vi "FitterParams.vi"(7 "eTestType":T1(ring), 8 "error in (no error)":errorcluster, 10 "SignalParams":dbl[][](array[numeric])) -> (0 "error out":errorcluster, 2 "FitterParams":dbl[](array[numeric]))   [LabVIEW 2018, in "AnalysisPlugins.lvlib" / "PmuAnalysis.lvclass"]
uses:
  PmuAnalysis.lvclass
  <vilib>/Utility/error.llb/Error Cluster From Error Code.vi
  <vilib>/ErrorRing/Error Ring.xnode
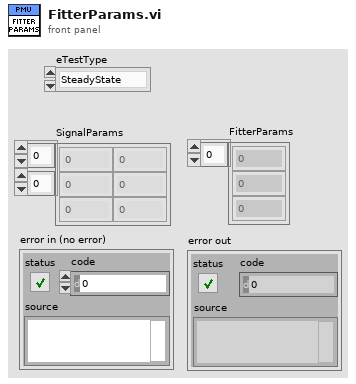
[diagram p1: front panel]
types:
  T1 = enum16{"SteadyState", "Modulation", "Ramp", "Step"}
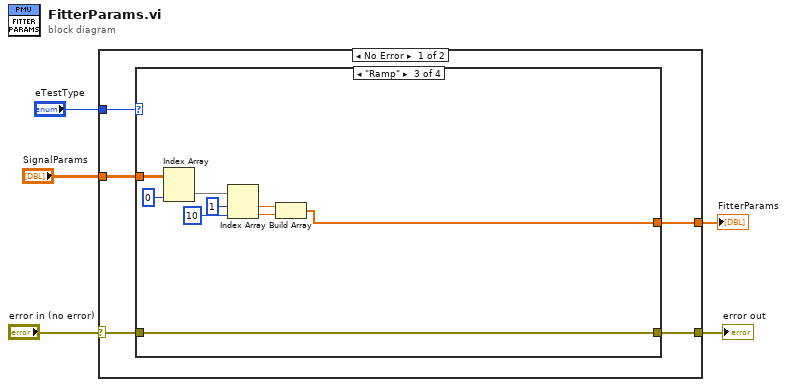
[diagram p0: block diagram]
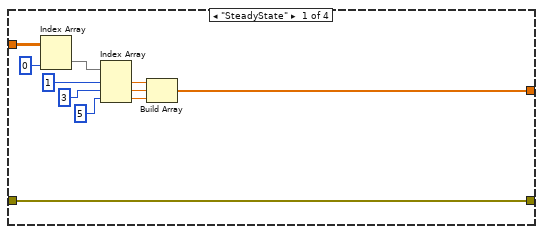
[diagram p2: hidden frame]
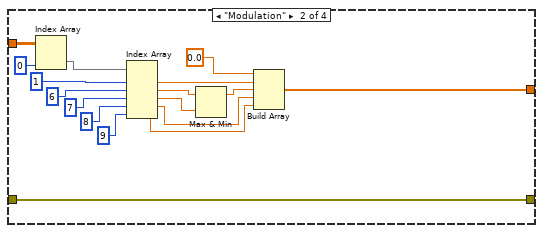
[diagram p3: hidden frame]
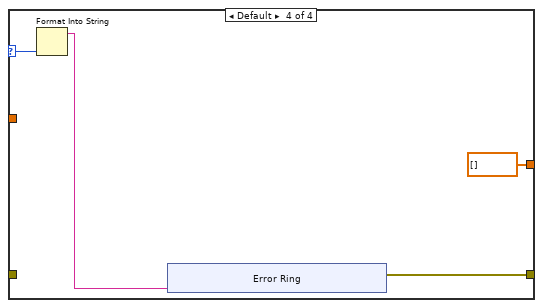
[diagram p4: hidden frame]
diagram:
  n1 = case shown="No Error" "error in (no error)" {
    selector: "error in (no error)" -> [w6 w59]
    tunnel: [w7 w59] -> w4
    tunnel: "eTestType" -> [w10 _]
    tunnel: "SignalParams" -> [w9 _]
    tunnel: [w8 _] -> w1
    frame No Error {
      n2 = case shown="\"Ramp\"" w10 {
        selector: w10 -> [_ _ _ w51]
        tunnel: w9 -> [w21 w38 w47 _]
        tunnel: [w12 w23 w40 dbl[] []] -> w8
        tunnel: [w11 w22 w39 w48] -> w7
        tunnel: w6 -> [w11 w22 w39 _]
        frame "SteadyState" {
          n3 = Index Array(array=w21, index (col)=0 ("disabled index (col)")) -> (element=w19:dbl[])  [unwired: 1 in]
          n4 = Index Array(array=w19, index #1=1 ("index"), index #2=3 ("index"), index #3=5 ("index")) -> (element #1=w15:dbl, element #2=w14:dbl, element #3=w13:dbl)
          n5 = Build Array(w15, w14, w13) -> (w12:dbl[])
        }
        frame "Modulation" {
          n6 = Index Array(array=w38, index (col)=0 ("disabled index (col)")) -> (element=w36:dbl[])  [unwired: 1 in]
          n7 = Index Array(array=w36, index #1=1 ("index"), index #2=6 ("index"), index #3=7 ("index"), index #4=8 ("index"), index #5=9 ("index")) -> (element #1=w29:dbl, element #2=w28:dbl, element #3=w27:dbl, element #4=w25:dbl, element #5=w24:dbl)
          n8 = Max & Min(x=w28, y=w27) -> (max(x,y)=w26:dbl)  [unwired: 1 out]
          n9 = Build Array(0.0 ("element"), w29, w26, w25, w24) -> (w23:dbl[])
        }
        frame "Ramp" {
          n10 = Index Array(array=w47, index (col)=0 ("disabled index (col)")) -> (element=w45:dbl[])  [unwired: 1 in]
          n11 = Index Array(array=w45, index #1=1 ("index"), index #2=10 ("index")) -> (element #1=w41:dbl, element #2=w42:dbl)
          n12 = Build Array(w41, w42) -> (w40:dbl[])
        }
        frame Default {
          n13 = Format Into String(w51) -> (resulting string=w50:string)  [unwired: 3 in, 1 out]
          n14 = xnode "Error Ring"("parameter 0"=w50) -> ("error out"=w48:errorcluster)
        }
      }
    }
    frame Error {
    }
  }
  "error out" <- w4
  "FitterParams" <- w1
